vi "ArrayFunctions_CheckForDups(I32).vi"(1 "Array":i32[](array[numeric])) -> (15 "DupElements":i32[](array[numeric]), 16 "DupElements(String)":string, 17 "FoundDups":bool)   [LabVIEW 2016]
doc: "Prüft ein Array auf Duplikate und gibt diese aus"
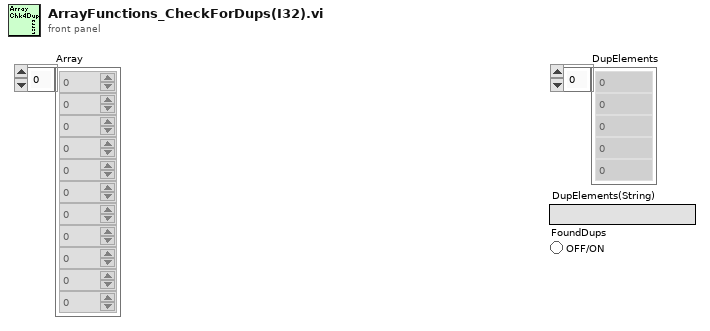
[diagram p1: front panel]
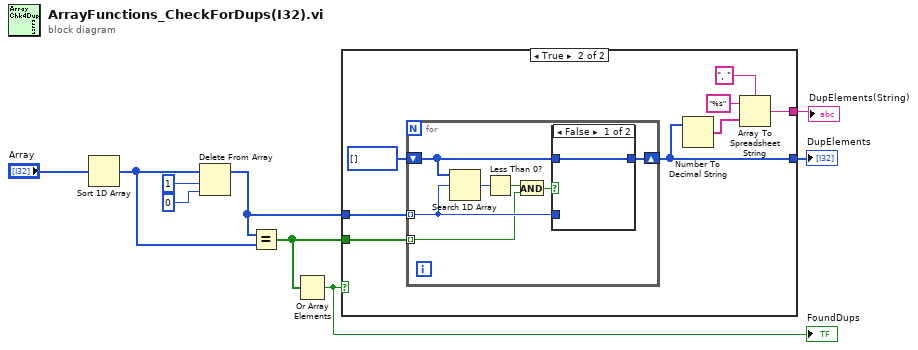
[diagram p0: block diagram]
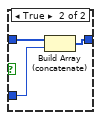
[diagram p3: hidden frame]
diagram:
  n1 = Sort 1D Array(array="Array") -> (sorted array=w2:i32[])
  n2 = Delete From Array(array=w2, length=1, index=0) -> (array with subset deleted=w7:i32[])  [unwired: 1 out]
  n3 = Equal?(x=w7, y=w2) -> (x = y?=w6:bool[])
  n4 = Or Array Elements(Boolean array=w6) -> (logical OR=w4:bool)
  "FoundDups" <- w4
  n5 = case shown="True" w4 {
    tunnel: w7 -> [_ w17]
    tunnel: w6 -> [_ w16]
    tunnel: [_ w11] -> w5
    tunnel: [_ w12] -> w1
    frame False {
    }
    frame True {
      n6 = for {
        tunnel: w17 -> [w22] mode=indexing
        tunnel: w16 -> [w18] mode=indexing
        shift-right: [w24] -> w11
        shift-left: i32[] [] ("array w/ subset deleted") -> [w23]
        n7 = Search 1D Array(1D array=w23, element=w22) -> (index of element=w21:i32)  [unwired: 1 in]
        n8 = Less Than 0?(x=w21) -> (x < 0?=w20:bool)
        n9 = And(x=w20, y=w18) -> (x .and. y?=w19:bool)
        n10 = case shown="False" w19 {
          tunnel: [w25 w28] -> w24
          tunnel: w23 -> [w25 w27]
          tunnel: w22 -> [_ w26]
          frame False {
          }
          frame True {
            n11 = Build Array (concatenate)(w27, w26) -> (w28:i32[])
          }
        }
      }
      n12 = Number To Decimal String(number=w11) -> (decimal integer string=w10:string[])  [unwired: 1 in]
      n13 = Array To Spreadsheet String(delimiter (Tab)=", ", array=w10, 3:"%s" ("format string")) -> (spreadsheet string=w12:string)
    }
  }
  "DupElements" <- w5
  "DupElements(String)" <- w1
